vi "TCP Write.vi"(11 "Message Queues out":T2) -> ()   [LabVIEW 2021, in "TCP Library.lvlib"]
uses:
  Lauda Integral XT-150 TCU/TCP Library.lvlib
  Main/Main Queue Cluster.ctl
  support/Message Queue/Message Cluster.ctl
  TCP Connection Settings.ctl
  TCP Multiple Connections State.ctl
  Tag VIs/Tag FGV Operation Enum.ctl
  support/Message Queue/Enqueue Message (Single).vi
  <vilib>/addons/_JKI.lib/Serialization/JSON/JKI JSON Serialization.lvlib
  Shared Variables/Dynamic Shared Variables.lvlib
  support/Message Queue/Message Queue.lvlib
panel:
  in  "TCP Settings In":T1={"address"="10.131.72.83", "port"=50023}
  in  "error in (no error)":errorcluster
  out "decimal integer string":string
  out "length":i32
  out "*(type *) &x":string
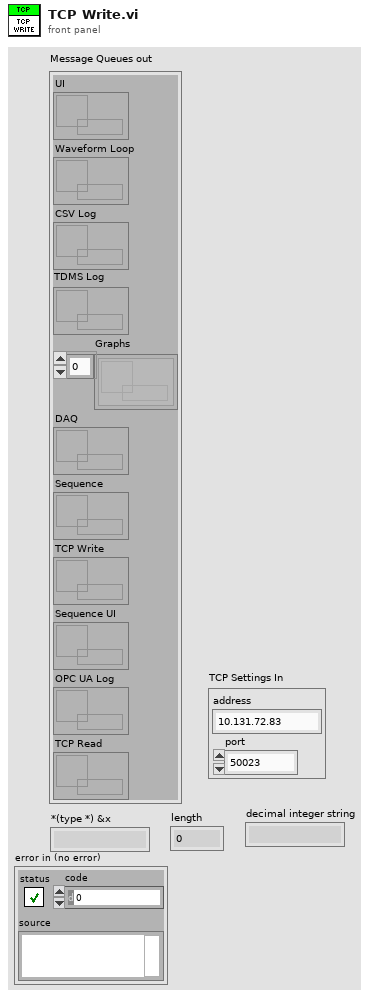
[diagram p1: front panel]
types:
  T1 = typedef "TCP Library.lvlib/TCP Connection Settings.ctl" = cluster{"address":string, "port":u16}
  T2 = typedef "Main Queue Cluster.ctl" = cluster{"UI":refnum<queue>, "Waveform Loop":refnum<queue>, "CSV Log":refnum<queue>, "TDMS Log":refnum<queue>, "Graphs":refnum<queue>[], "DAQ":refnum<queue>, "Sequence":refnum<queue>, "TCP Write":refnum<queue>, "Sequence UI":refnum<queue>, "OPC UA Log":refnum<queue>, "TCP Read":refnum<queue>}
  T3 = typedef "TCP Library.lvlib/TCP Multiple Connections State.ctl" = enum16{"Initialize", "Status Check", "Send Data", "Stop"}
  T4 = cluster{"listener ID":refnum<k5>, "State":T3, "Clients":refnum<k5>[], "ELN Number":string}
  T5 = typedef "Tag FGV Operation Enum.ctl" = enum16{"Init", "Set Notification Queue", "Create Tag", "Commit", "Write Tag (Numeric)", "Write Tag (Boolean)", "Read All Tags", "Read One Tag", "Delete Tag Category", "Set Alarm Parameters (Numeric)", "Set Alarm Parameters (Boolean)", "Enable All Alarms", "Disable All Alarms", "Delete All Tags", "Read Alarms", "Ack Alarm", "Read Alarm Parameters (Numeric)", "Read Alarm Parameters (Boolean)"}
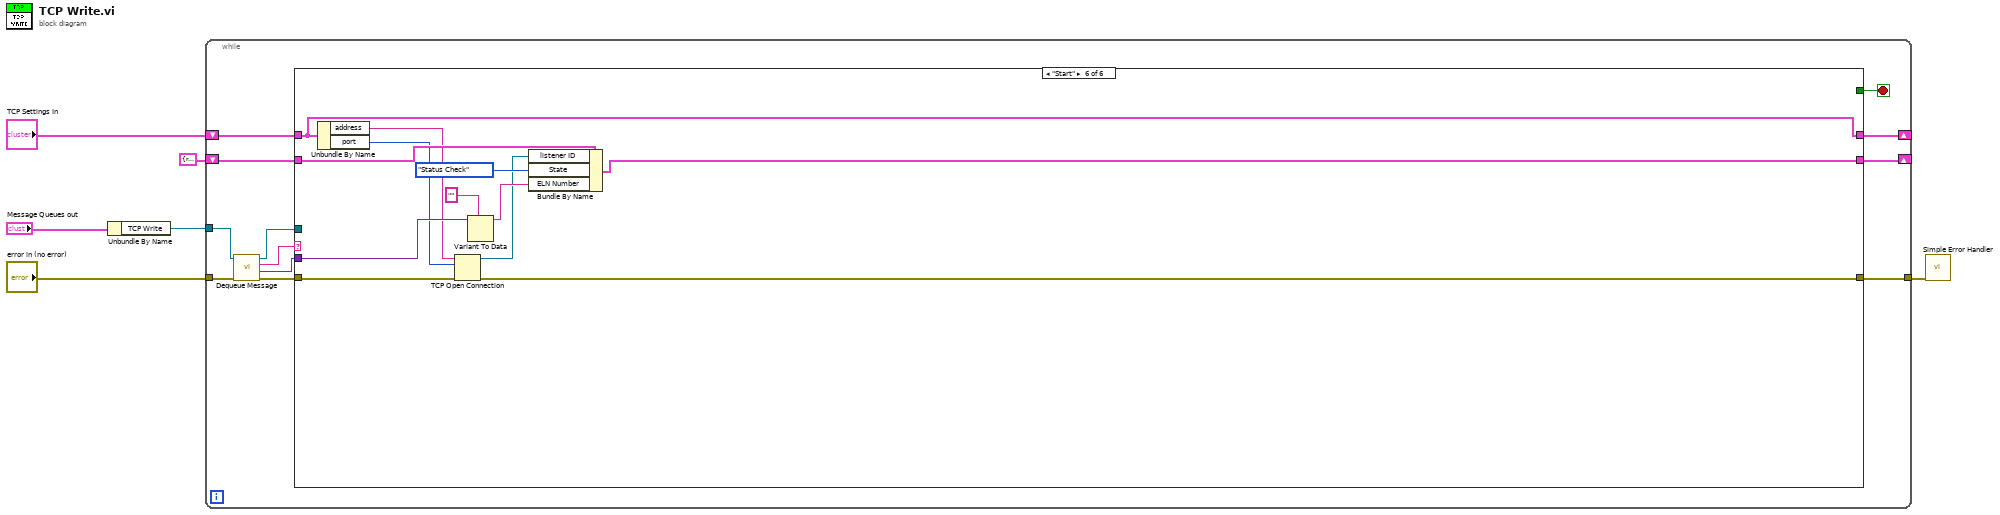
[diagram p0: block diagram]
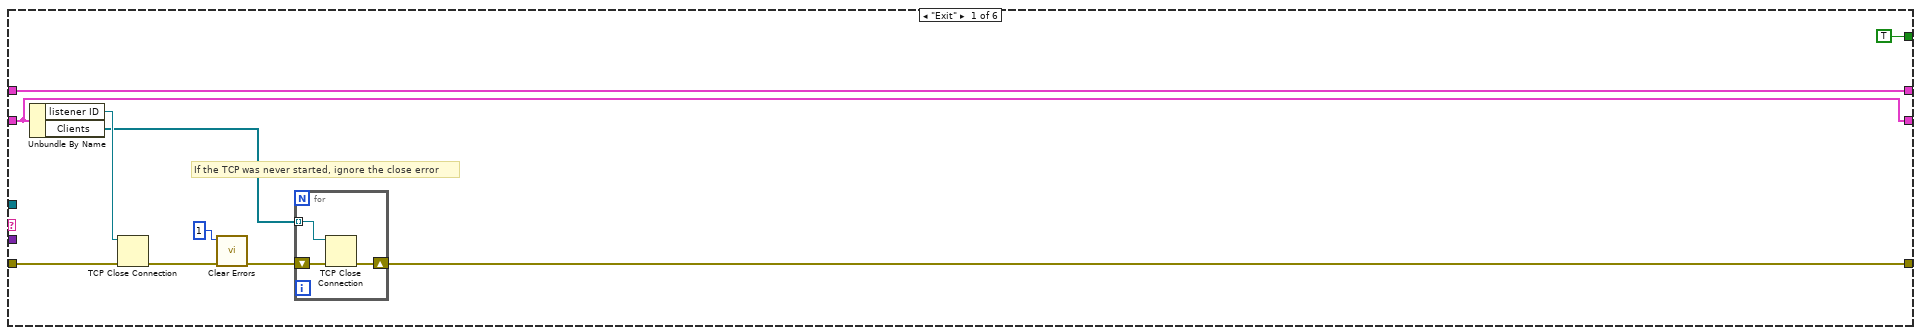
[diagram p2: hidden frame]
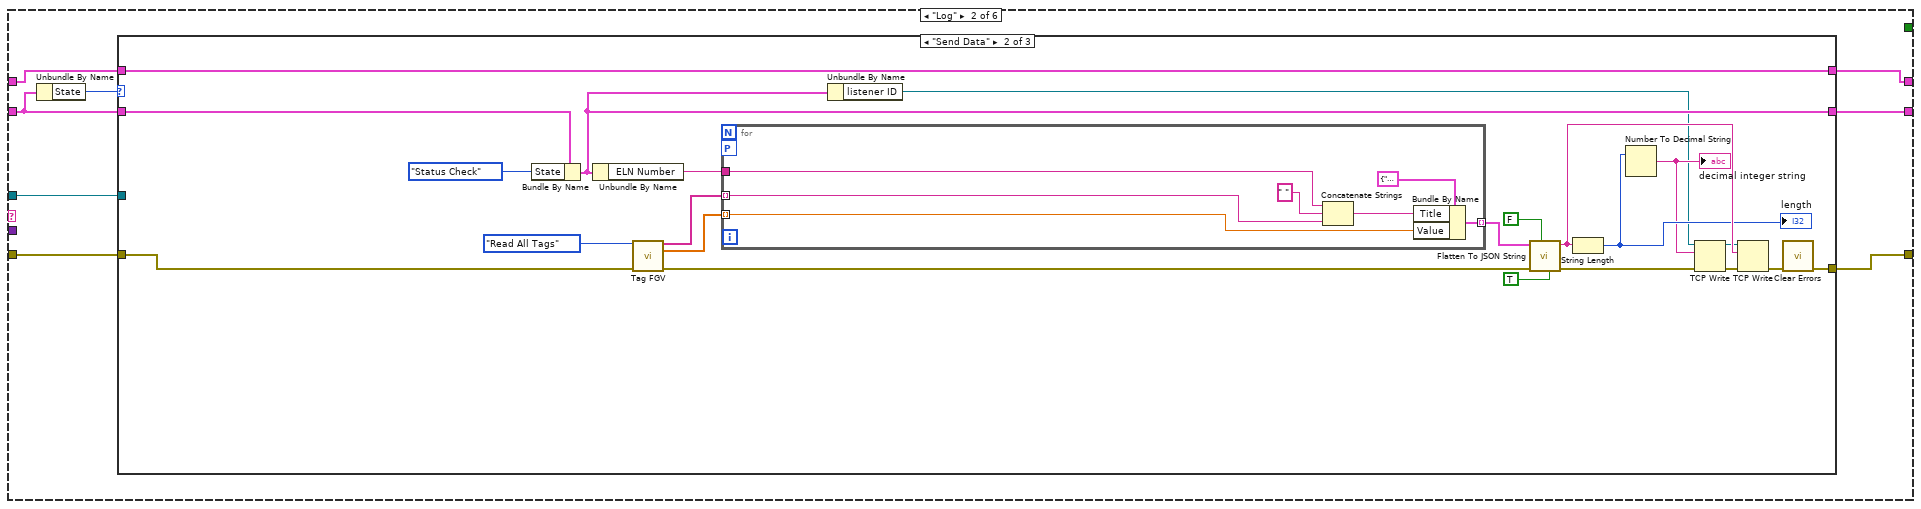
[diagram p3: hidden frame]
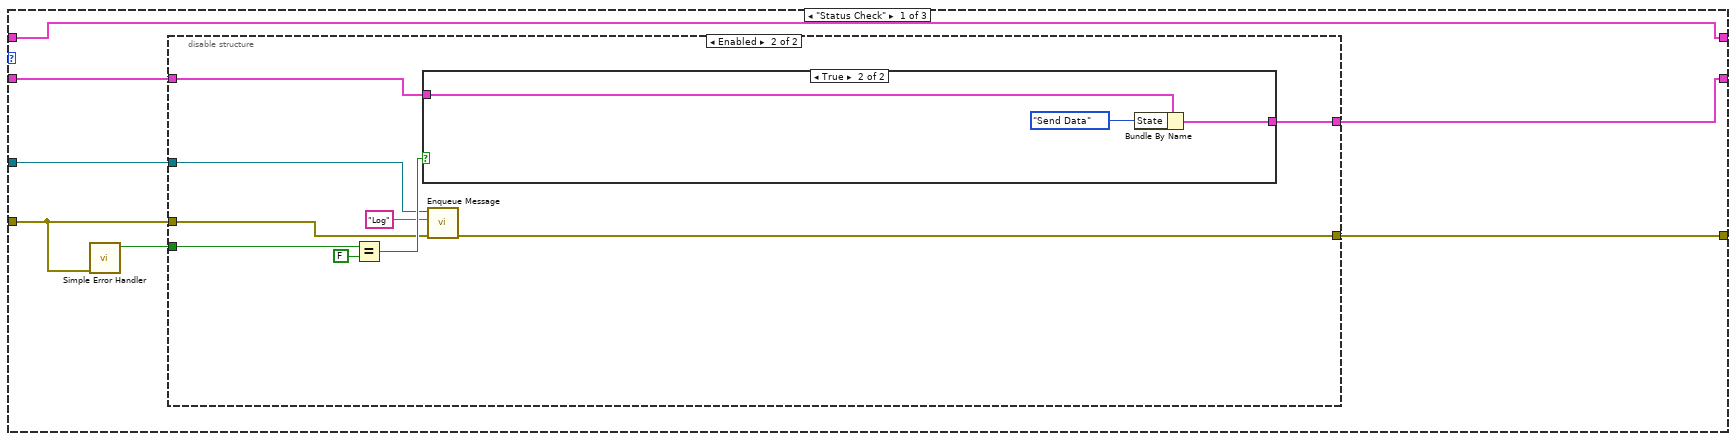
[diagram p4: hidden frame]
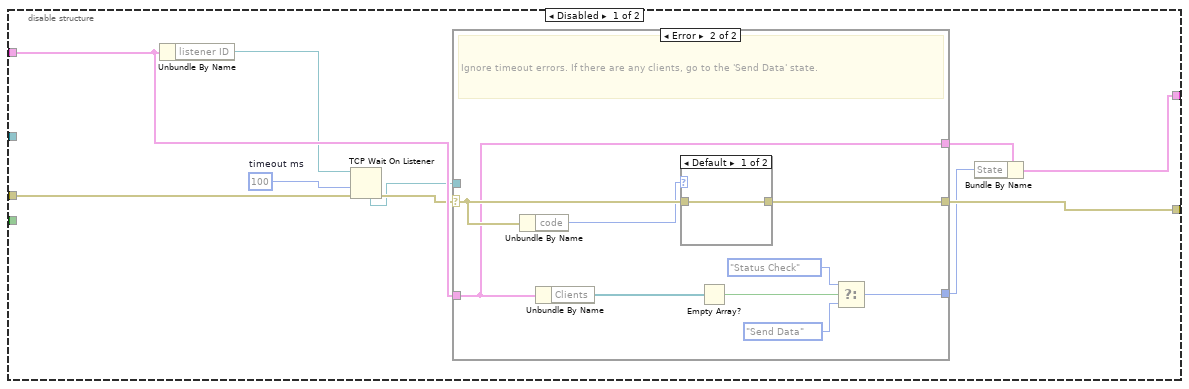
[diagram p5: hidden frame]
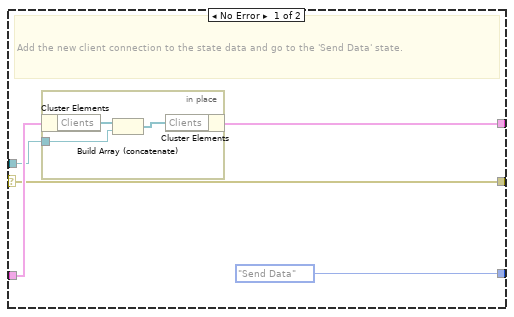
[diagram p6: hidden frame]
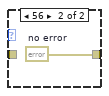
[diagram p7: hidden frame]
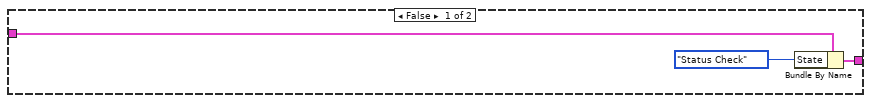
[diagram p8: hidden frame]
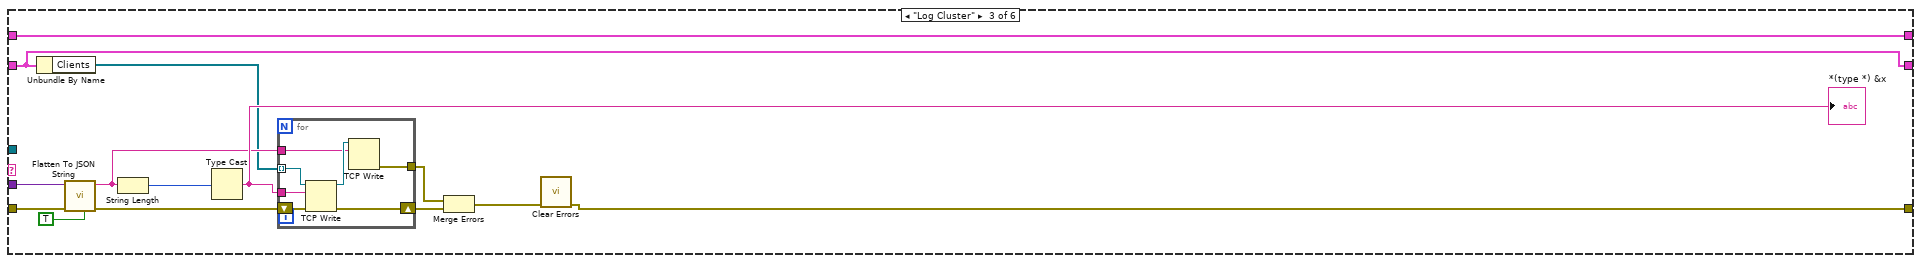
[diagram p10: hidden frame]
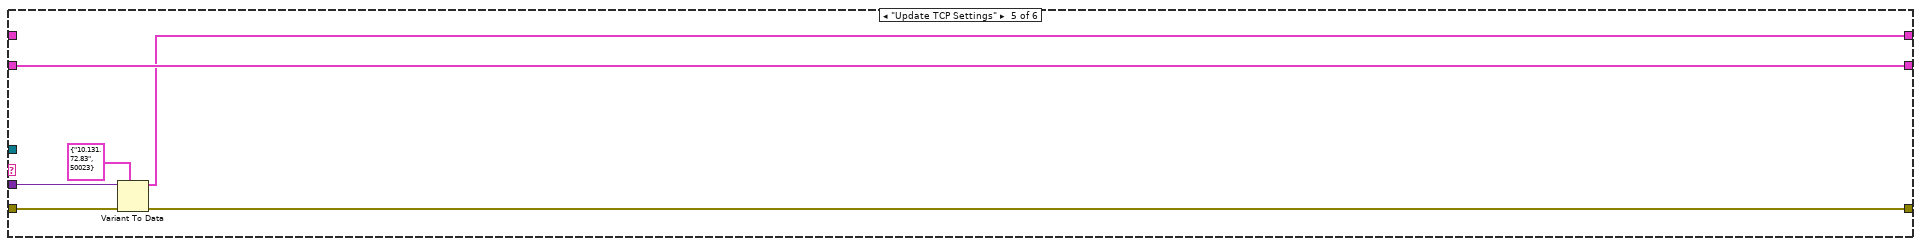
[diagram p12: hidden frame]
diagram:
  n1 = Unbundle By Name("Message Queues out") -> ("TCP Write"=w5:refnum<queue>)
  n2 = while {
    tunnel: w5 -> [w16]
    shift-right: [w13] -> _
    shift-left: T4 {"listener ID"=refnum, "State"=enum."Initialize", "Clients"=[], "ELN Number"=""} -> [w12]
    tunnel: [w11] -> w3
    tunnel: "error in (no error)" -> [w10]
    shift-right: [w8] -> _
    shift-left: "TCP Settings In" -> [w7]
    stop <- w15 stop-if-true
    n3 = call "Dequeue Message.vi"("error in (no error)"=w10, "Message Queue"=w16) -> ("error out"=w17:errorcluster, "Message Data"=w14:variant, "Message"=w18:string, "dup Message Queue"=w9:refnum<queue>)  [unwired: 6 in]
    n4 = case shown="\"Start\"" w18 {
      tunnel: w17 -> [w28 w39 w128 w145 w148 w156]
      tunnel: [TRUE _ _ _ _ _] -> w15
      tunnel: w14 -> [_ _ w127 _ w149 w160]
      tunnel: [w23 w36 w124 w146 w151 w162] -> w13
      tunnel: w12 -> [w23 w37 w124 w146 w151 w163]
      tunnel: [w24 w35 w126 w145 w148 w155] -> w11
      tunnel: w9 -> [_ w34 _ _ _ _]
      tunnel: [w19 w33 w123 w144 w147 w154] -> w8
      tunnel: w7 -> [w19 w32 w123 w144 _ w154]
      frame "Exit" {
        # "If the TCP was never started, ignore the close error"
        n5 = Unbundle By Name(w23) -> ("listener ID"=w26:refnum<k5>, "Clients"=w25:refnum<k5>[])
        n6 = TCP Close Connection(connection ID=w26, error in (no error)=w28) -> (error out=w22:errorcluster)  [unwired: 1 in, 1 out]
        n7 = call <vilib>:"Clear Errors.vi"("error in (no error)"=w22, "specific error code to clear (0: all)"=1) -> ("error out"=w21:errorcluster)  [unwired: 4 in, 1 out]
        n8 = for {
          shift-right: [w30] -> w24
          shift-left: w21 -> [w31]
          tunnel: w25 -> [w29] mode=indexing
          n9 = TCP Close Connection(connection ID=w29, error in (no error)=w31) -> (error out=w30:errorcluster)  [unwired: 1 in, 1 out]
        }
      }
      frame "Log" {
        n10 = Unbundle By Name(w37) -> ("State"=w38:T3)
        n11 = case shown="\"Send Data\"" w38 {
          tunnel: w39 -> [w43 w112 w121]
          tunnel: w37 -> [w46 w103 w122]
          tunnel: [w44 w96 w122] -> w36
          tunnel: [w45 w101 w121] -> w35
          tunnel: w34 -> [w41 _ _]
          tunnel: [w40 w91 w120] -> w33
          tunnel: w32 -> [w40 w91 w120]
          frame "Status Check" {
            n12 = call <vilib>:"Simple Error Handler.vi"("error in (no error)"=w43) -> ("error?"=w42:bool)  [unwired: 4 in, 4 out]
            n13 = disable-structure shown="Enabled" {
              disable-tunnel: w46 -> [w56 w82]
              disable-tunnel: [w55 w76] -> w45
              disable-tunnel: [w48 w81] -> w44
              disable-tunnel: w43 -> [w47 w77]
              disable-tunnel: w42 -> [_ w83]
              disable-tunnel: w41 -> [_ w79]
              frame Disabled {
                w54 = 100  # timeout ms
                n14 = Unbundle By Name(w56) -> ("listener ID"=w51:refnum<k5>)
                n15 = TCP Wait On Listener(8:w47, 9:w54, 11:w51) -> (0:w53:errorcluster, 4:w52:refnum<k5>)  [unwired: 4 out]
                n16 = case shown="Error" w53 {
                  selector: w53 -> [w59 w73]
                  tunnel: [TCP_Multiple_Connections_State."Send Data" ("States") w67] -> w49
                  tunnel: w52 -> [w60 _]
                  tunnel: w56 -> [w61 w70]
                  tunnel: [w58 w70] -> w50
                  tunnel: [w59 w71] -> w55
                  frame No Error {
                    # "Add the new client connection to the state data and go to the 'Send Data' state."
                    n17 = in-place {
                      in-place-border: w60 -> [w62]
                      n18 = in-place-cluster #1(w61) -> ("Clients"=w64:refnum<k5>[])
                      n19 = Build Array (concatenate)(w64, w62) -> (w63:refnum<k5>[])
                      n20 = in-place-cluster #1("Clients"=w63) -> (w58:T4)
                    }
                  }
                  frame Error {
                    # "Ignore timeout errors. If there are any clients, go to the 'Send Data' state."
                    n21 = Unbundle By Name(w73) -> ("code"=w72:i32)
                    n22 = Unbundle By Name(w70) -> ("Clients"=w69:refnum<k5>[])
                    n23 = case shown="Default" w72 {
                      tunnel: w73 -> [w74 _]
                      tunnel: [w74 w75] -> w71
                      frame Default {
                      }
                      frame 56 {
                        w75 = errorcluster {"status"=FALSE, "code"=0, "source"=""}  # no error
                      }
                    }
                    n24 = Empty Array?(array=w69) -> (empty?=w68:bool)
                    n25 = Select(t=TCP_Multiple_Connections_State."Status Check" ("States"), s=w68, f=TCP_Multiple_Connections_State."Send Data" ("States")) -> (s? t:f=w67:T3)
                  }
                }
                n26 = Bundle By Name(cluster=w50, "State"=w49) -> (w48:T4)
              }
              frame Enabled {
                n27 = Equal?(x=w83, y=FALSE) -> (x = y?=w80:bool)
                n28 = case shown="True" w80 {
                  tunnel: w82 -> [w85 w90]
                  tunnel: [w86 w89] -> w81
                  frame False {
                    n29 = Bundle By Name(cluster=w85, "State"=TCP_Multiple_Connections_State."Status Check") -> (w86:T4)
                  }
                  frame True {
                    n30 = Bundle By Name(cluster=w90, "State"=TCP_Multiple_Connections_State."Send Data") -> (w89:T4)
                  }
                }
                n31 = call-poly "Enqueue Message.vi"("error in (no error)"=w77, "Message"="Log", "Message Queue"=w79) -> ("error out"=w76:errorcluster)  [unwired: 7 in, 1 out]
              }
            }
          }
          frame "Send Data" {
            n32 = Bundle By Name(cluster=w103, "State"=TCP_Multiple_Connections_State."Status Check" ("Initial State")) -> (w96:T4)
            n33 = Unbundle By Name(w96) -> ("ELN Number"=w100:string)
            n34 = call "Tag FGV.vi"("Operation"=Tag_FGV_Operation_Enum."Read All Tags", "error in (no error)"=w112) -> ("Tag Names"=w108:string[], "Tag Values"=w107:dbl[], "error out"=w105:errorcluster)  [unwired: 6 in, 5 out]
            n35 = for {
              tunnel: w108 -> [w116] mode=indexing
              tunnel: w107 -> [w118] mode=indexing
              tunnel: [w117] -> w106 mode=indexing
              tunnel: w100 -> [w114]
              workers-P: _ -> [_]
              n36 = Concatenate Strings(w114, " " ("string"), w116) -> (w115:string)
              n37 = Bundle By Name(cluster=cluster{"Title":string, "Value":dbl} {"Title"="", "Value"=0.0}, "Title"=w115, "Value"=w118) -> (w117:cluster{"Title":string, "Value":dbl})
            }
            n38 = Unbundle By Name(w96) -> ("listener ID"=w95:refnum<k5>)
            n39 = call <vilib>:"Flatten To JSON String.vi"("Enums As String (F)"=TRUE, "Multiline (T)"=FALSE, "error in (no error)"=w105, "Variant"=w106) -> ("error out"=w104:errorcluster, "JSON String"=w111:string)  [unwired: 6 in]
            n40 = String Length(string=w111) -> (length=w99:i32)
            "length" <- w99
            n41 = Number To Decimal String(number=w99) -> (decimal integer string=w98:string)  [unwired: 1 in]
            "decimal integer string" <- w98
            n42 = TCP Write(connection ID=w95, data in=w98, error in (no error)=w104) -> (connection ID out=w97:refnum<k5>, error out=w94:errorcluster)  [unwired: 2 out]
            n43 = TCP Write(connection ID=w97, data in=w111, error in (no error)=w94) -> (error out=w93:errorcluster)  [unwired: 3 out]
            n44 = call <vilib>:"Clear Errors.vi"("error in (no error)"=w93) -> ("error out"=w101:errorcluster)  [unwired: 5 in, 1 out]
          }
          frame Default {
          }
        }
      }
      frame "Log Cluster" {
        n45 = Unbundle By Name(w124) -> ("Clients"=w125:refnum<k5>[])
        n46 = call <vilib>:"Flatten To JSON String.vi"("Enums As String (F)"=TRUE, "error in (no error)"=w128, "Variant"=w127) -> ("error out"=w129:errorcluster, "JSON String"=w133:string)  [unwired: 7 in]
        n47 = String Length(string=w133) -> (length=w135:i32)
        n48 = Type Cast(x=w135) -> (*(type *) &x=w134:string)  [unwired: 1 out]
        "*(type *) &x" <- w134
        n49 = for {
          tunnel: w134 -> [w142]
          tunnel: w133 -> [w141]
          tunnel: [w140] -> w131
          shift-right: [w139] -> w130
          shift-left: w129 -> [w138]
          tunnel: w125 -> [w137] mode=indexing
          n50 = TCP Write(connection ID=w137, data in=w142, error in (no error)=w138) -> (connection ID out=w143:refnum<k5>, error out=w139:errorcluster)  [unwired: 2 out]
          n51 = TCP Write(connection ID=w143, data in=w141) -> (error out=w140:errorcluster)  [unwired: 1 in, 3 out]
        }
        n52 = Merge Errors(w131, w130) -> (w132:errorcluster)
        n53 = call <vilib>:"Clear Errors.vi"("error in (no error)"=w132) -> ("error out"=w126:errorcluster)  [unwired: 5 in, 1 out]
      }
      frame Default {
      }
      frame "Update TCP Settings" {
        n54 = Variant To Data(error in=w148, type=T1 {"address"="10.131.72.83", "port"=50023} ("TCP Settings In 2"), Variant=w149) -> (data=w147:T1)  [unwired: 1 out]
      }
      frame "Start" {
        n55 = Unbundle By Name(w154) -> ("address"=w153:string, "port"=w152:u16)
        n56 = TCP Open Connection(address=w153, remote port or service name=w152, error in (no error)=w156) -> (connection ID=w157:refnum<k5>, error out=w155:errorcluster)  [unwired: 2 in]
        n57 = Variant To Data(type="", Variant=w160) -> (data=w158:string)  [unwired: 1 in, 1 out]
        n58 = Bundle By Name(cluster=w163, "listener ID"=w157, "State"=TCP_Multiple_Connections_State."Status Check" ("Initial State"), "ELN Number"=w158) -> (w162:T4)
      }
    }
  }
  n59 = call <vilib>:"Simple Error Handler.vi"("error in (no error)"=w3) -> ()  [unwired: 4 in, 5 out]
